vi "ReadEdvrRef.vi"(8 "error in (no error)":errorcluster, 11 "EdvrObject in":refnum<class "EdvrObject.lvclass">) -> (0 "error out":errorcluster, 2 "Edvr":T1, 3 "EdvrObject out":refnum<class "EdvrObject.lvclass">)   [LabVIEW 2020, in "OpenLvVision_OpenCv.lvlib" / "EdvrObject.lvclass"]
uses:
  EdvrObject.lvclass
  TypeDef/Edvr.ctl
  EdvrObject.lvclass/EdvrObject.ctl
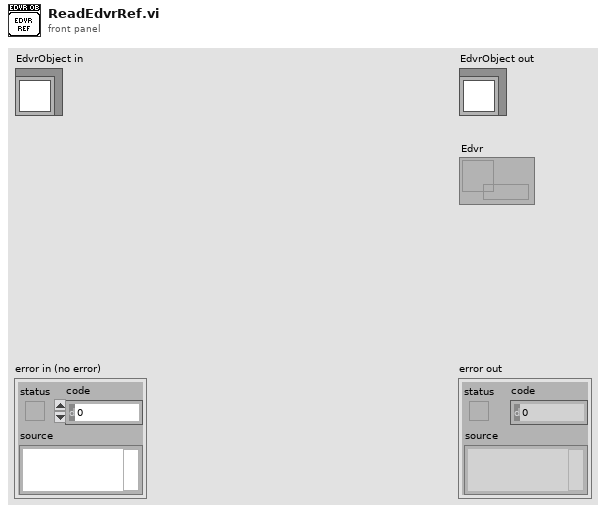
[diagram p1: front panel]
types:
  T1 = typedef "OpenLvVision_OpenCv.lvlib/EdvrObject.lvclass/Edvr.ctl" = refnum<data-value>
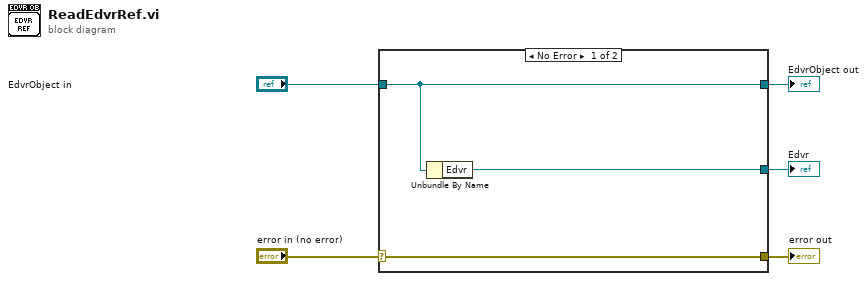
[diagram p0: block diagram]
diagram:
  n1 = case shown="No Error" "error in (no error)" {
    selector: "error in (no error)" -> [w8 w9]
    tunnel: [w8 w9] -> w4
    tunnel: [w7 w10] -> w2
    tunnel: "EdvrObject in" -> [w7 w10]
    tunnel: [w6 _] -> w1
    frame No Error {
      n2 = Unbundle By Name(w7) -> ("Edvr"=w6:T1)
    }
    frame Error {
    }
  }
  "error out" <- w4
  "EdvrObject out" <- w2
  "Edvr" <- w1
